vi "分割影像.vi"() -> ()   [LabVIEW 2015]
uses:
  <vilib>/vision/Image Controls.llb/IMAQ Image.ctl
panel:
  in  "Bias":cluster{"Width":i32, "Height":i32}
  in  "size":cluster{"Width":i32, "Height":i32}={"Width"=32, "Height"=32}
  out "Array":T1[][](array[plugin-control])
  in  "interval":cluster{"Width":i32, "Height":i32}={"Width"=37, "Height"=0}
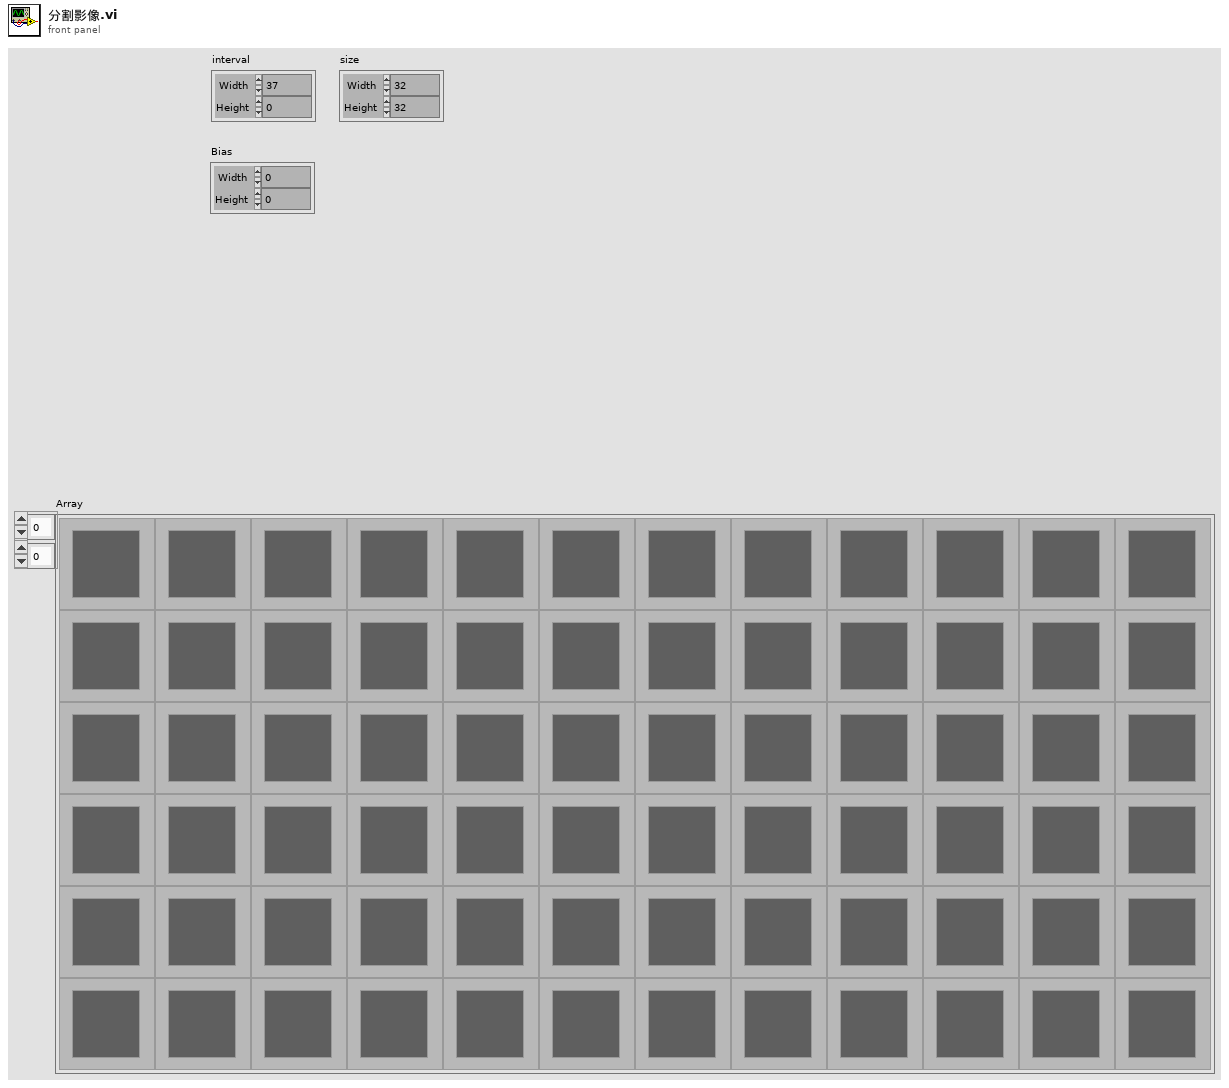
[diagram p1: front panel]
types:
  T1 = typedef "IMAQ Image.ctl" = refnum<image>
  T2 = cluster{"Width":i32, "Height":i32, i32, i32, dbl}
  T3 = typedef "ROI Descriptor" = cluster{"Global Rectangle":i32[], "Contours":cluster{"ID":enum32{"External", "Internal"}, "Type":u32, "Coordinates":i32[]}[]}
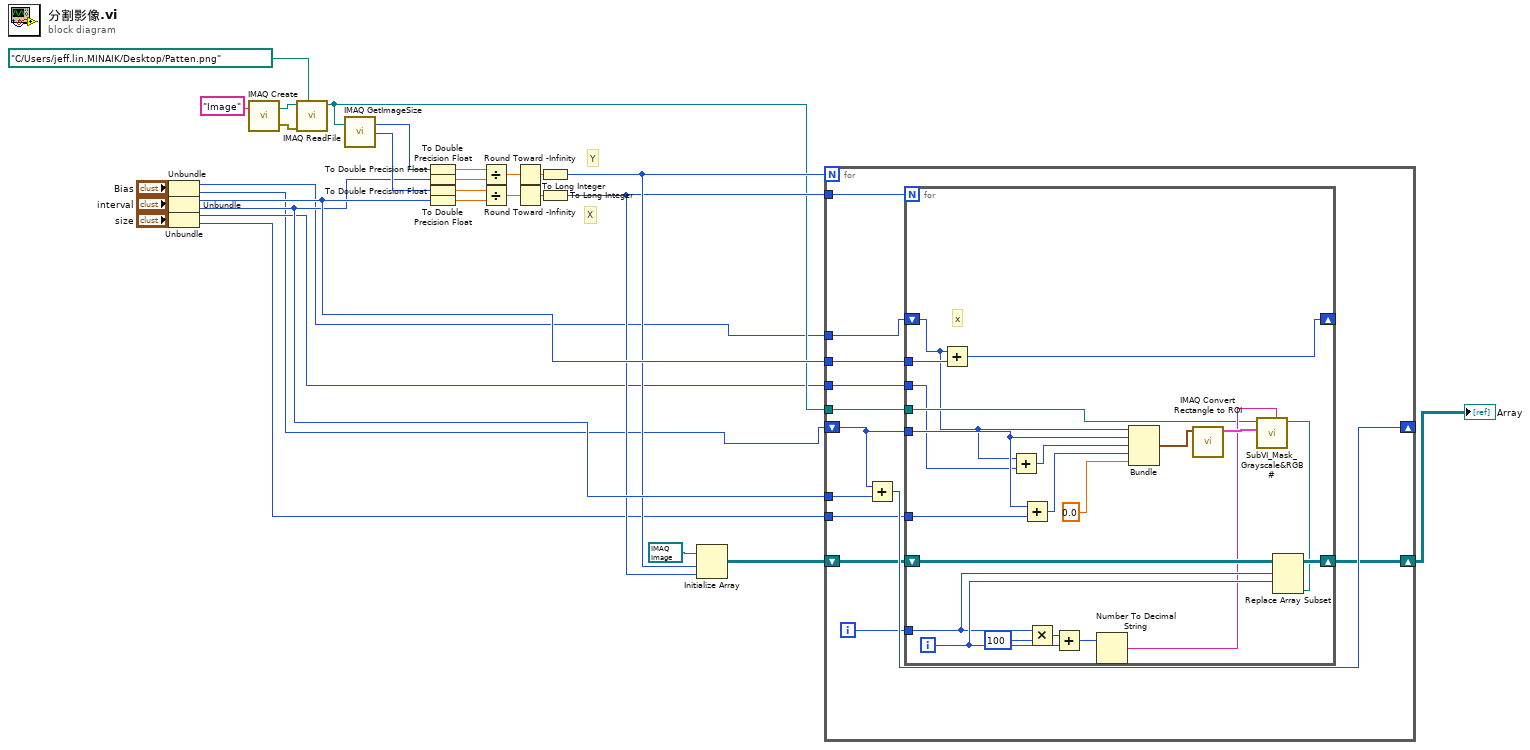
[diagram p0: block diagram]
diagram:
  # "Y"
  # "X"
  n1 = Unbundle("Bias") -> ("Width"=w2:i32, "Height"=w1:i32)
  n2 = Unbundle("interval") -> ("Width"=w14:i32, "Height"=w13:i32)
  n3 = Unbundle("size") -> ("Width"=w6:i32, "Height"=w5:i32)
  n4 = call "IMAQ Create"("Image Name"="Image") -> ("New Image"=w27:T1, "error out"=w28:errorcluster)  [unwired: 4 in]
  n5 = call "IMAQ ReadFile"("File Path"=path "C:/Users/jeff.lin.MINAIK/Desktop/Patten.png", "error in (no error)"=w28, "Image"=w27) -> ("Image Out"=w7:T1)  [unwired: 4 in, 4 out]
  n6 = call "IMAQ GetImageSize"("Image"=w7) -> ("Y Resolution"=w20:i32, "X Resolution"=w24:i32)  [unwired: 3 in, 1 out]
  n7 = To Double Precision Float(number=w20) -> (double precision float=w19:dbl)
  n8 = To Double Precision Float(number=w13) -> (double precision float=w15:dbl)
  n9 = To Double Precision Float(number=w24) -> (double precision float=w23:dbl)
  n10 = To Double Precision Float(number=w14) -> (double precision float=w16:dbl)
  n11 = Divide(x=w19, y=w15) -> (x/y=w17:dbl)
  n12 = Divide(x=w23, y=w16) -> (x/y=w22:dbl)
  n13 = Round Toward -Infinity(1:w17) -> (0:w18:dbl)
  n14 = Round Toward -Infinity(1:w22) -> (0:w21:dbl)
  n15 = To Long Integer(number=w18) -> (32bit integer=w11:i32)
  n16 = To Long Integer(number=w21) -> (32bit integer=w10:i32)
  n17 = Initialize Array(T1 refnum ("Image Dst Out"), w11, w10) -> (w9:T1[][])
  n18 = for {
    N: w11 -> [_]
    tunnel: w10 -> [w41]
    shift-right: [w39] -> _
    shift-left: w1 -> [w30]
    tunnel: w14 -> [w40]
    tunnel: w13 -> [w38]
    shift-right: [w36] -> w8
    shift-left: w9 -> [w35]
    tunnel: w7 -> [w34]
    tunnel: w6 -> [w33]
    tunnel: w5 -> [w32]
    tunnel: w2 -> [w31]
    i -> [w37]
    n19 = Add(x=w30, y=w38) -> (x+y=w39:i32)
    n20 = for {
      N: w41 -> [_]
      tunnel: w30 -> [w58]
      shift-right: [w61] -> _
      shift-left: w31 -> [w42]
      tunnel: w40 -> [w43]
      tunnel: w32 -> [w57]
      tunnel: w37 -> [w47]
      shift-right: [w54] -> w36
      shift-left: w35 -> [w55]
      tunnel: w34 -> [w45]
      tunnel: w33 -> [w44]
      i -> [w50]
      # "x"
      n21 = Add(x=w42, y=w43) -> (x+y=w61:i32)
      n22 = Add(x=w42, y=w44) -> (x+y=w60:i32)
      n23 = Add(x=w58, y=w57) -> (x+y=w59:i32)
      n24 = Multiply(x=w47, y=100) -> (x*y=w49:i32)
      n25 = Add(x=w49, y=w50) -> (x+y=w48:i32)
      n26 = Number To Decimal String(number=w48) -> (decimal integer string=w46:string)  [unwired: 1 in]
      n27 = Bundle("Width"=w42, "Height"=w58, w60, w59, 0.0) -> (w56:T2)  [unwired: 1 in]
      n28 = call "IMAQ Convert Rectangle to ROI"("Rectangle"=w56) -> ("ROI Descriptor"=w53:T3)  [unwired: 8 in, 1 out]
      n29 = call "SubVI_Mask_Grayscale&RGB #.vi"("Image Register Name"=w46, "ROI Descriptor"=w53, "Image Src In"=w45) -> ("Image Dst Out"=w52:T1)  [unwired: 5 in, 3 out]
      n30 = Replace Array Subset(array=w55, new element=w52, index (row)=w47, index (col)=w50) -> (w54:T1[][])
    }
  }
  "Array" <- w8
